vi "5p1_HW_Task2_fishele.vi"() -> ()   [LabVIEW 2021]
panel:
  out "Min or Max?":string="Both are equal to 0"
  in  "f''":dbl
  in  "f'":dbl
  # "Test for Max or Min Based on First and Second Derivative"
  # "Input"
  # "Output"
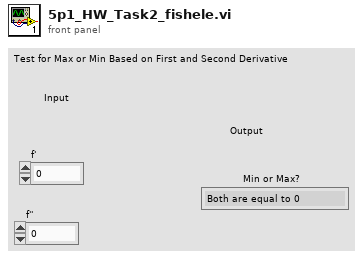
[diagram p1: front panel]
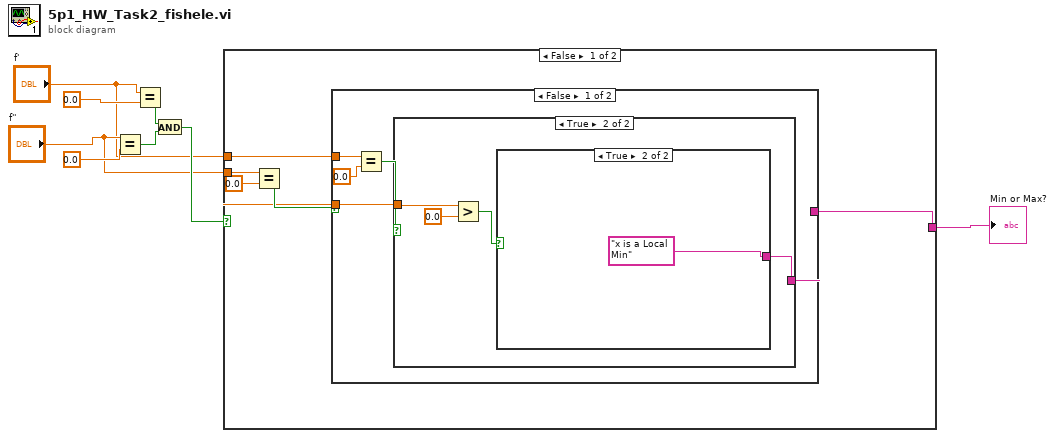
[diagram p0: block diagram]
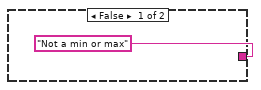
[diagram p2: hidden frame]
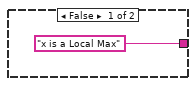
[diagram p3: hidden frame]
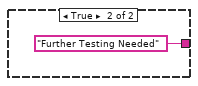
[diagram p4: hidden frame]
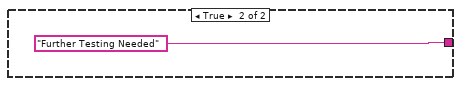
[diagram p5: hidden frame]
diagram:
  n1 = Equal?(x="f''", y=0.0) -> (x = y?=w4:bool)
  n2 = Equal?(x="f'", y=0.0) -> (x = y?=w5:bool)
  n3 = And(x=w5, y=w4) -> (x .and. y?=w3:bool)
  n4 = case shown="False" w3 {
    tunnel: [w11 "Further Testing Needed"] -> w8
    tunnel: "f''" -> [w9 _]
    tunnel: "f'" -> [w10 _]
    frame False {
      n5 = Equal?(x=w9, y=0.0) -> (x = y?=w12:bool)
      n6 = case shown="False" w12 {
        tunnel: [w18 "Further Testing Needed"] -> w11
        tunnel: w10 -> [w17 _]
        tunnel: w9 -> [w14 _]
        frame False {
          n7 = Equal?(x=w17, y=0.0) -> (x = y?=w15:bool)
          n8 = case shown="True" w15 {
            tunnel: ["Not a min or max" w20] -> w18
            tunnel: w14 -> [_ w23]
            frame False {
            }
            frame True {
              n9 = Greater?(x=w23, y=0.0) -> (0:w21:bool)
              n10 = case shown="True" w21 {
                tunnel: ["x is a Local Max" "x is a Local Min"] -> w20
                frame False {
                }
                frame True {
                }
              }
            }
          }
        }
        frame True {
        }
      }
    }
    frame True {
    }
  }
  "Min or Max?" <- w8
